vi "Write Weight Slot.vi"(8 "error in (no error)":errorcluster, 9 "Weight Slot":T1, 10 "weight slot":i32, 11 "WorkTable Class in":refnum<class "WorkTable Class.lvclass">) -> (0 "error out":errorcluster, 3 "WorkTable Class out":refnum<class "WorkTable Class.lvclass">)   [LabVIEW 2011, in "WorkTable Class.lvclass"]
uses:
  WorkTable Class.lvclass
  Type Definitions/Worktable_Weight.ctl
  Vec3d Class/Vec3d Class.lvclass
  Orient3d Class/Orient3d Class.lvclass
  Config Manager Class/Type Definitions/Weight Type.ctl
  Utils/Type Definitions/Position_Orientation.ctl
  WorkTable Class.lvclass/WorkTable Class.ctl
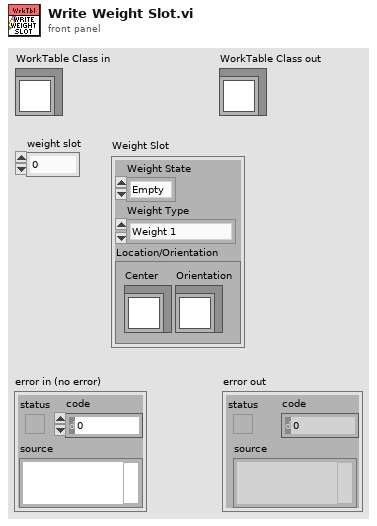
[diagram p1: front panel]
types:
  T1 = typedef "Worktable_Weight.ctl" = cluster{"Weight State":enum16{"Empty", "Populated"}, "Weight Type":T2, "Location/Orientation":T3}
  T2 = typedef "Weight Type.ctl" = enum16{"Weight 1", "Weight 2", "Weight 3", "Weight 4", "Weight 5", "Weight 6", "Weight 7", "Weight 8"}
  T3 = typedef "Position_Orientation.ctl" = cluster{"Center":refnum<class "Vec3d Class.lvclass">, "Orientation":refnum<class "Orient3d Class.lvclass">}
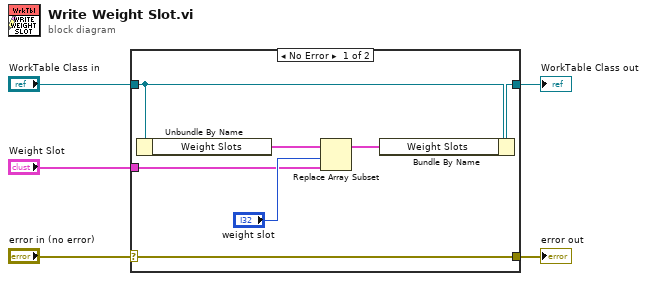
[diagram p0: block diagram]
diagram:
  n1 = case shown="No Error" "error in (no error)" {
    selector: "error in (no error)" -> [w12 w13]
    tunnel: [w12 w13] -> w4
    tunnel: [w11 w14] -> w2
    tunnel: "WorkTable Class in" -> [w10 w14]
    tunnel: "Weight Slot" -> [w6 _]
    frame No Error {
      n2 = Unbundle By Name(w10) -> ("Weight Slots"=w9:T1[])
      n3 = Replace Array Subset(array=w9, new element=w6, index="weight slot") -> (w8:T1[])
      n4 = Bundle By Name(cluster=w10, "Weight Slots"=w8) -> (w11:refnum<class "WorkTable Class.lvclass">)
    }
    frame Error {
    }
  }
  "error out" <- w4
  "WorkTable Class out" <- w2
